vi "001_ZLG_CAN.vi"(11 "Queue Ref":T1={"UI"=refnum, "Message"=refnum, "Data"=refnum, "Caller"=refnum, "Name"="000 Common", "Data Path"=path "D:/NBT/01-Project/02-Processing/NBT-TestPlatform V2/NBT-TestPlatform V2.0.3/Config/NBT/NBT_V1.0.0/Project/0001_HZKD_ST01/00_DataSource/001_PLC/01_PLC", "Class Path"=path "", "SubPanel"=refnum, "Project Name"="", "MNT"="", "Title"="", "Data Source"=refnum, "Queue List"={}, "VI"=refnum, "UE"=refnum}) -> ()   [LabVIEW 2020]
doc: "001_ZLG_CAN.vi"
uses:
  Alin/QMH/000 Module Data Type.ctl
  Alin/QMH/Queue Message.ctl
  9999 SubVI/Global/Data Global/SDQ Data Type.ctl
  002 Driver/005 CAN/ZLG/ZLG_CAN_Channel.ctl
  002 Driver/005 CAN/ZLG/ZLG CAN.ctl
  002 Driver/005 CAN/ZLG/XNET_ZLG CAN/SubVIs/CAN/data_type/ZCAN_Transmit_Data.ctl
  <vilib>/Utility/miscctls.llb/LVMapReplaceAction.ctl
  002 Driver/005 CAN/ZLG/XNET_ZLG CAN/SubVIs/CAN/data_type/ZCAN_InitCAN_setting_CANET.ctl
  ba99fbad-406a-44a4-8ea9-c630dc189d5e.vi
  <vilib>/Utility/config.llb/Read Key (String).vi
  <vilib>/Utility/config.llb/Write Key (String).vi
  <vilib>/Utility/file.llb/Read Delimited Spreadsheet (string).vi
  <vilib>/Utility/file.llb/Write Delimited Spreadsheet (string).vi
  <vilib>/Utility/config.llb/NI_LVConfig.lvlib
panel:
  out "Name":string
  in  "Data Load":bool
  in  "ID":string(combo)
  out "Open":bool
  out "Read Delay(ms)":u32
  out "Write Delay(ms)":u32
  in  "Input":string
  in  "CAN Enable":bool
  out "Read":string[][](table) caption="单体电压排序(降序)"
  in  "Start Frame":u32=112 format="0x%08x"
  in  "Demo":string="{\"TIRC101_SV\":25.3,\"WorkMode_SV\":true}"
  in  "Multiple Parameter":string="{\"TIRC101_SV\":25.3,\"WorkMode_SV\":true}"
  in  "Write Test":bool
  out "Write Test":string[][](table) caption="单体电压排序(降序)"
  out "Write":string[][](table) caption="单体电压排序(降序)"
  out "Receive Frame":string
  out "Error":string
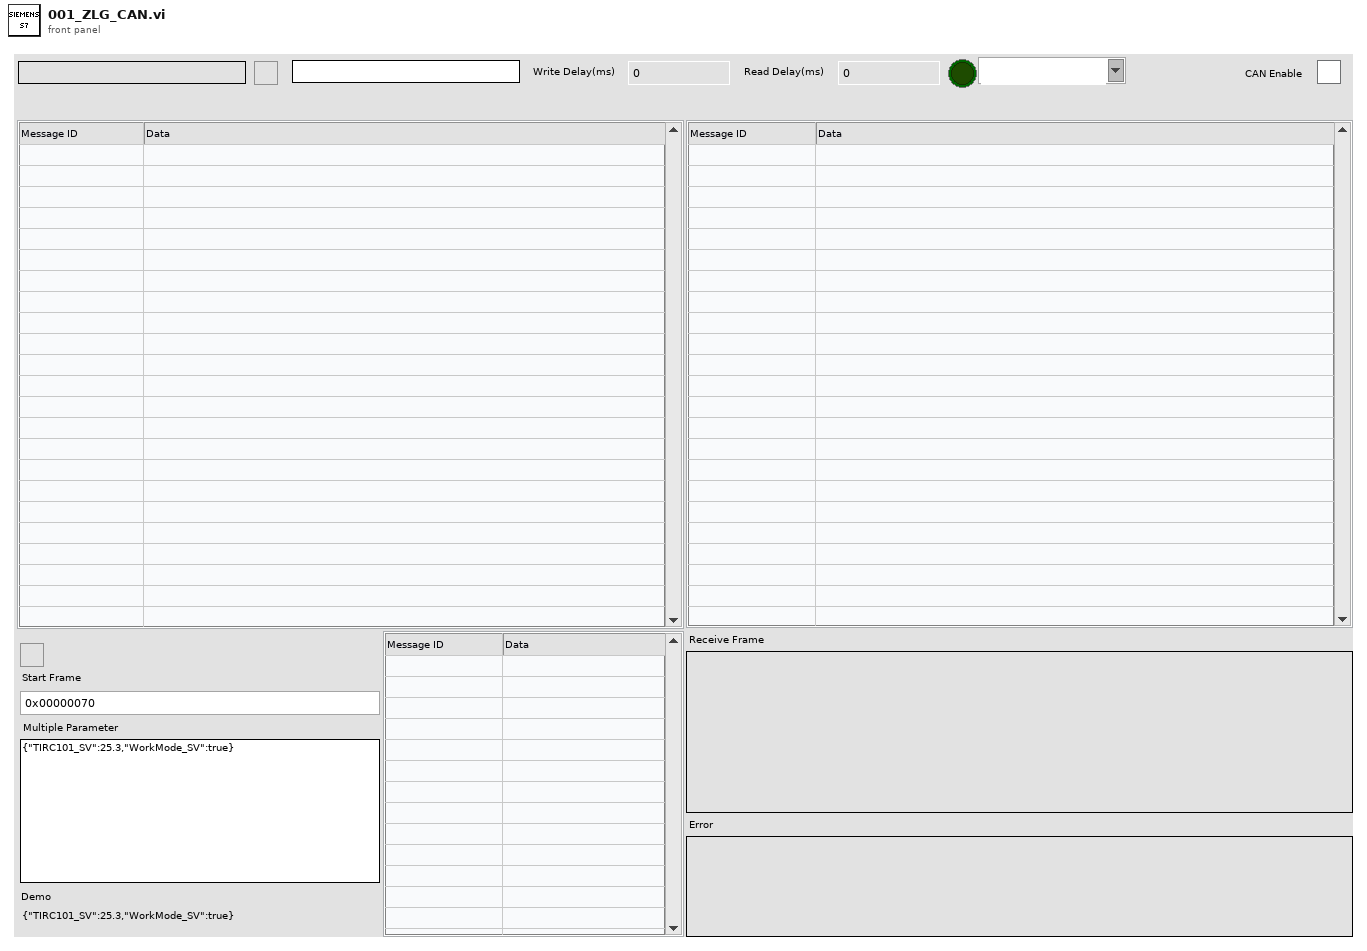
[diagram p1: front panel]
types:
  T1 = typedef "000 Module Data Type.ctl" = cluster{"UI":refnum<queue>, "Message":refnum<queue>, "Data":refnum<queue>, "Caller":refnum<queue>, "Name":string, "Data Path":path, "Class Path":path, "SubPanel":refnum<vi>, "Project Name":string, "MNT":string, "Title":string, "Data Source":refnum<queue>, "Queue List":map{string, refnum<queue>}, "VI":refnum<vi>, "UE":refnum<user-event>}
  T2 = typedef "SDQ Data Type.ctl" = cluster{"CAN Length":string, "CAN Name":string, "CAN ID":string, "CAN Type":string, "Test Item":string, "Byte Order":string, "Instruction":string, "Control Type":string, "Group":string, "Offset":dbl, "Coefficient":dbl, "Write Enable":bool, "Lable Type":string, "Key?":string, "Set Value":string, "Upper":dbl, "Lower":dbl, "Unit":string, "Formula":string, "Test Item Type":string, "Length":i32, "Address":string, "Name":string, "Identifier":string, "Data Type":string, "Enumerate?":string, "Enumerate List":string, "Data":string, "Source":string}
  T3 = typedef "ZLG_CAN_Channel.ctl" = cluster{"ChannelRef":u32, "DeviceRef":u32, "Reserved":u32, "CANModel":u32, "Index":u32, "CANChannel":u32, "TCPMode":u32, "LocalPort":u32, "RemotePort":u32, "IP":string, "Read?":bool, "Write?":bool}
  T4 = typedef "ZLG CAN.ctl" = cluster{"ID":string, "Name":string, "Length":i32, "Type":string, "Unit":string, "Upper":sgl, "Lower":sgl, "Set":i32, "Write Enable":bool, "Group":string, "Read Name":string, "CAN Fram Type":string, "CAN Message ID":string, "CAN Message Name":string, "CAN Byte Offset":i32, "CAN Bit Offset":i32, "CAN Message Length":i32, "Data":string}
  T5 = typedef "ZCAN_Transmit_Data.ctl" = cluster{"帧类型":u32, "帧格式":u32, "ID":u32, "数据长度":u8, "DATA":cluster{"CAN数据[0]":u8, "CAN数据[1]":u8, "CAN数据[2]":u8, "CAN数据[3]":u8, "CAN数据[4]":u8, "CAN数据[5]":u8, "CAN数据[6]":u8, "CAN数据[7]":u8}, "发送方式":u32}
  T6 = cluster{"Read Data":map{string, string}, "Open?":bool, "Queue Ref":T1, "Data":map{string, T2}, "Data List":T2[], "All Data":string[][], "Element":T2, "Title":string[], "Type":map{string, string}, "CAN":T3, "Delay":cluster{"Count Time(ms)":u32, "Delay Time(ms)":u32, "Next":string}, "CAN Data":map{string, T4}, "CAN Fram":map{string, map{string, T4}}, "ZCAN_Transmit_Data":T5, "CAN Element":u8[], "CAN Enable":bool, "dll Path":path}
  T7 = typedef "LVMapReplaceAction.ctl" = enum32{"Modify Entry only if found", "Add or Modify Entry", "Delete Entry"}
  T8 = typedef "ZCAN_InitCAN_setting_CANET.ctl" = cluster{"tcp_type":u32, "work_port":u32, "local_port":u32, "IP":string}
  T9 = typedef "NI_LVConfig.lvlib/Config Data RefNum.ctl" = refnum<k1>
  T10 = cluster{"Name":string, "Type":map{string, string}}
  T11 = cluster{u32, u8, u8, u8, u8, cluster{"[0]":u8, "[1]":u8, "[2]":u8, "[3]":u8, "[4]":u8, "[5]":u8, "[6]":u8, "[7]":u8}, u64}[]
  T12 = cluster{"CAN Element[0]":u8, "CAN Element[1]":u8, "CAN Element[2]":u8, "CAN Element[3]":u8, "CAN Element[4]":u8, "CAN Element[5]":u8, "CAN Element[6]":u8, "CAN Element[7]":u8}
  T13 = cluster{"CAN数据[0]":u8, "CAN数据[1]":u8, "CAN数据[2]":u8, "CAN数据[3]":u8, "CAN数据[4]":u8, "CAN数据[5]":u8, "CAN数据[6]":u8, "CAN数据[7]":u8}
  T14 = cluster{u32, "数据长度":u8, u8, u8, u8, "DATA":cluster{"CAN数据[0]":u8, "CAN数据[1]":u8, "CAN数据[2]":u8, "CAN数据[3]":u8, "CAN数据[4]":u8, "CAN数据[5]":u8, "CAN数据[6]":u8, "CAN数据[7]":u8}, "发送方式":u32}
  T15 = typedef "eventvkey.ctl" = enum16{"ASCII", "Enter", "Return", "Shift", "Ctrl", "Alt", "Cmd", "Opt", "Caps", "NumLock", "Clear", "Break", "Up", "Down", "Left", "Right", "Insert", "Delete", "Home", "End", "PageUp", "PageDown", "Escape", "Help", "Pause", "ScrollLock", "F1", "F2", "F3", "F4", "F5", "F6", "F7", "F8", "F9", "F10", "F11", "F12", "F13", "F14", "F15", "F16", "F17", "F18", "F19", "F20", "F21", "F22", "F23", "F24", "Play", "VolumeUp", "VolumeDown", "Mute", "Two Byte Char"}
  T16 = cluster{"Shift":bool, "Ctrl":bool, "Alt":bool, "Cmd":bool, "Opt":bool}
  T17 = cluster{"Queue List":map{string, refnum<queue>}, "Active Panel":string, "Queue":T1, "Active Row":i32, "All Data":string[][]}
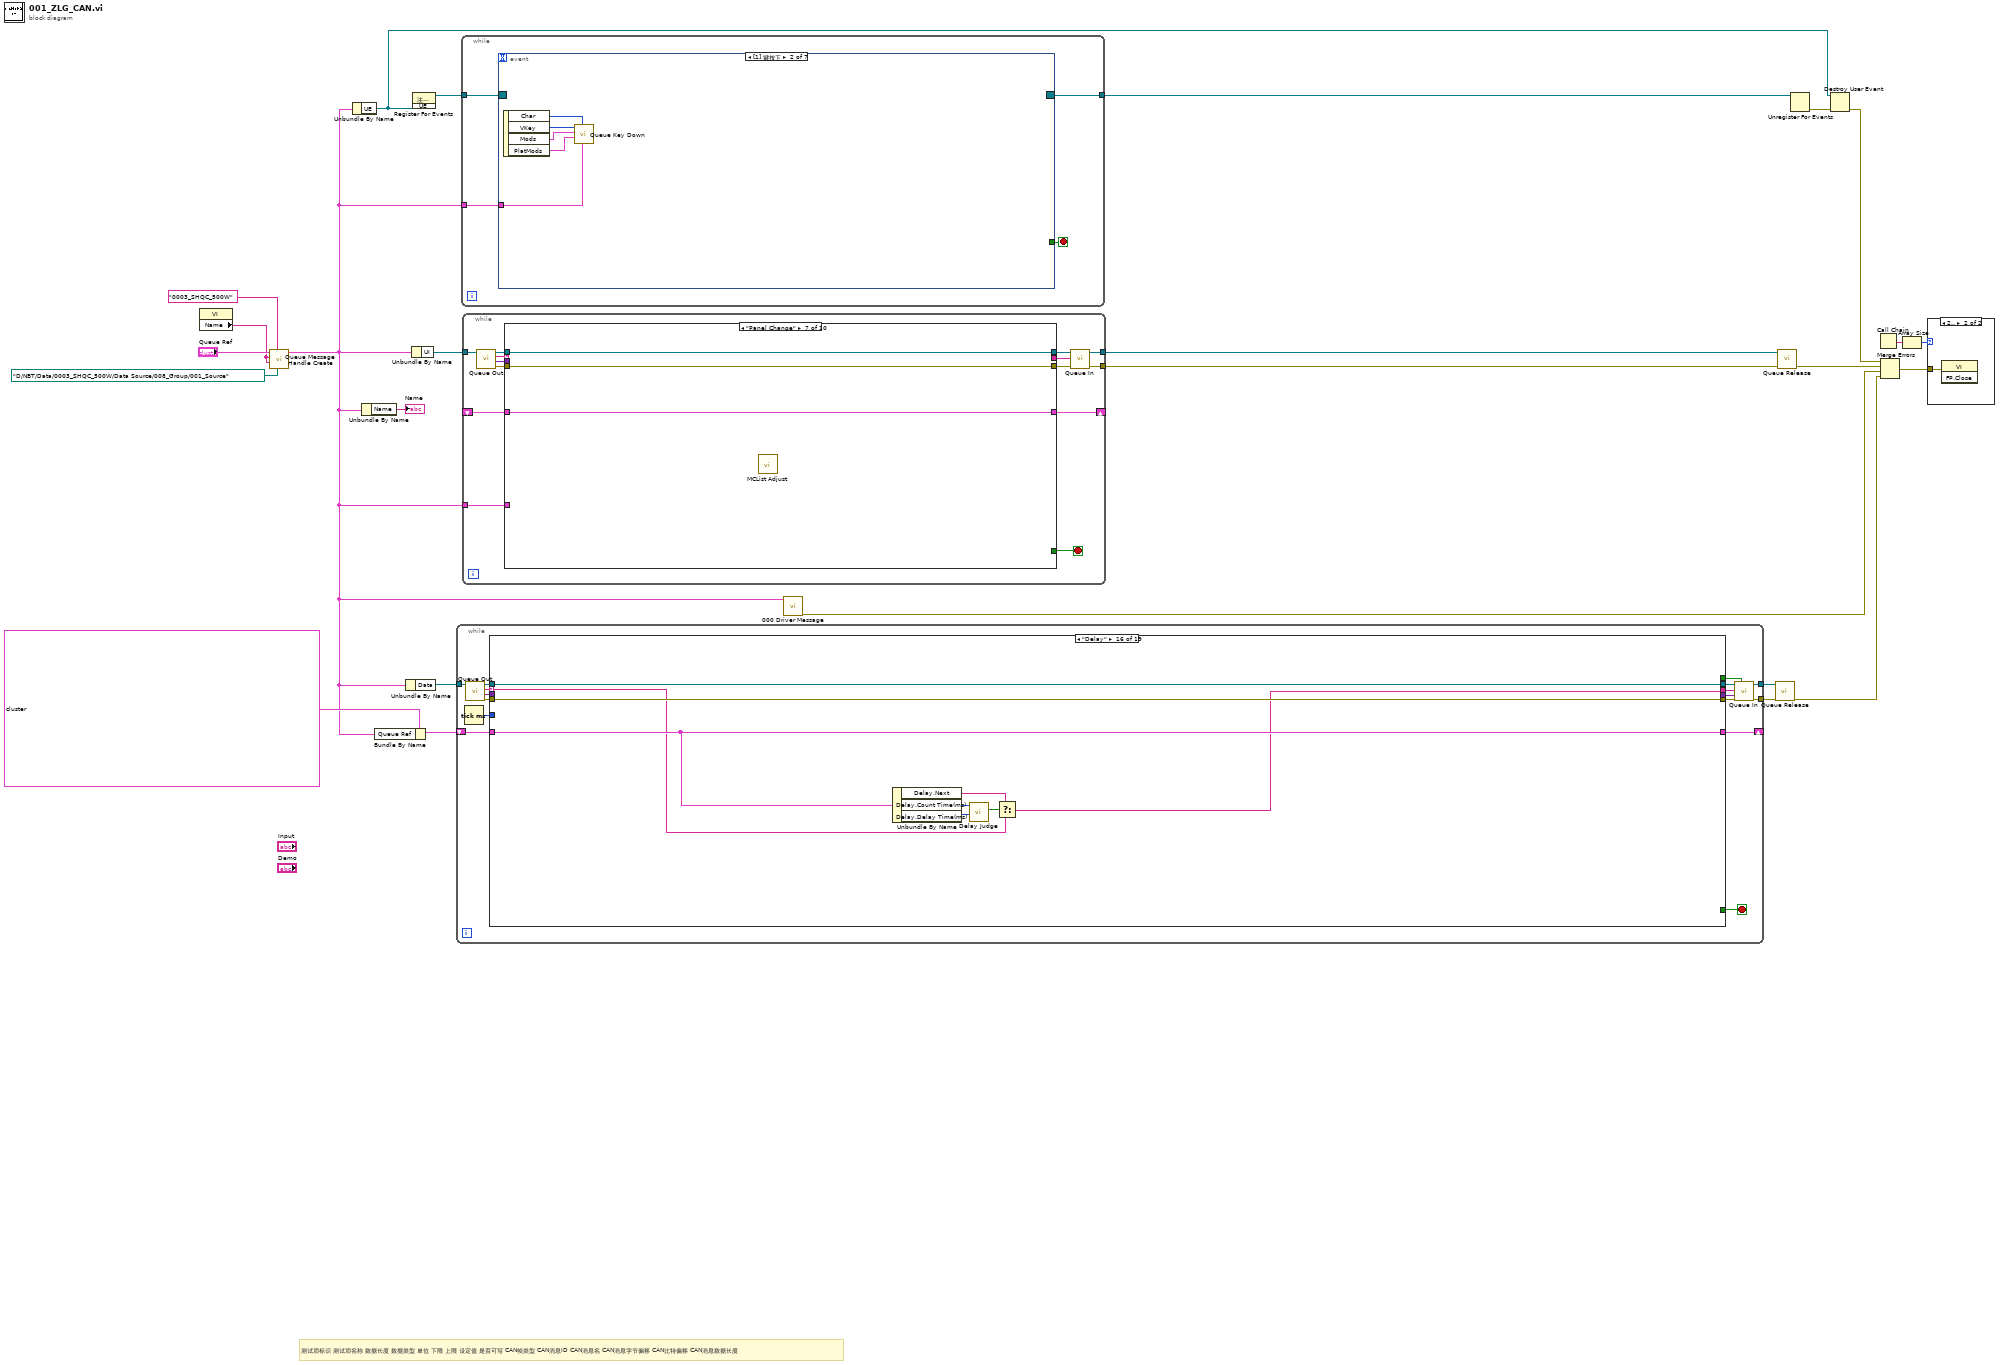
[diagram p0: block diagram]
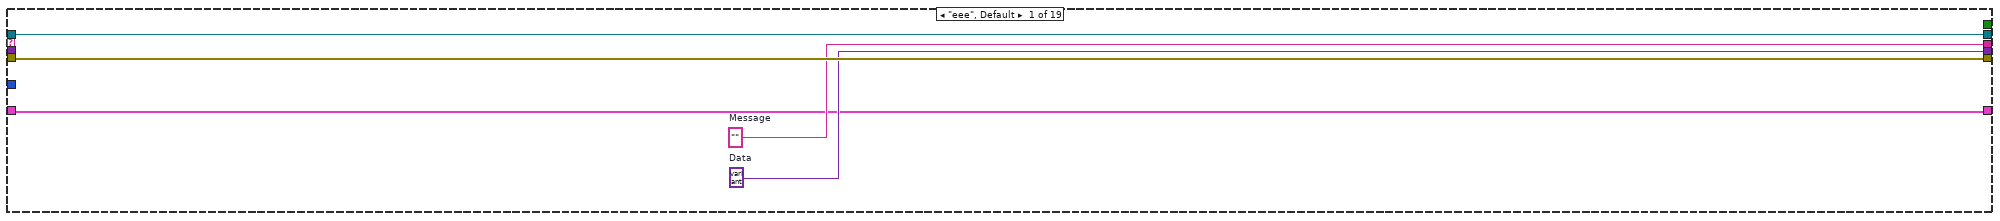
[diagram p2: hidden frame]
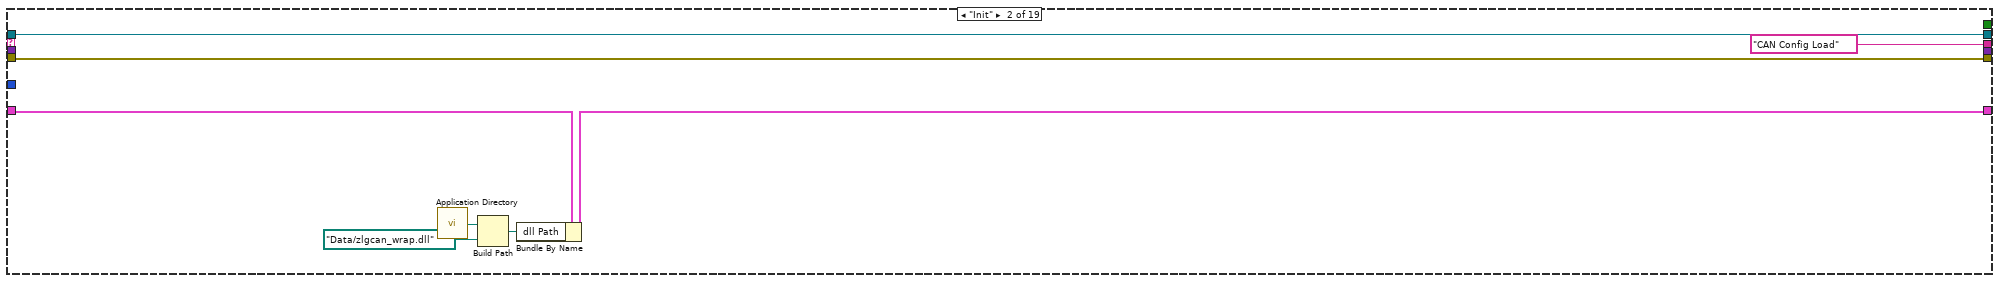
[diagram p3: hidden frame]
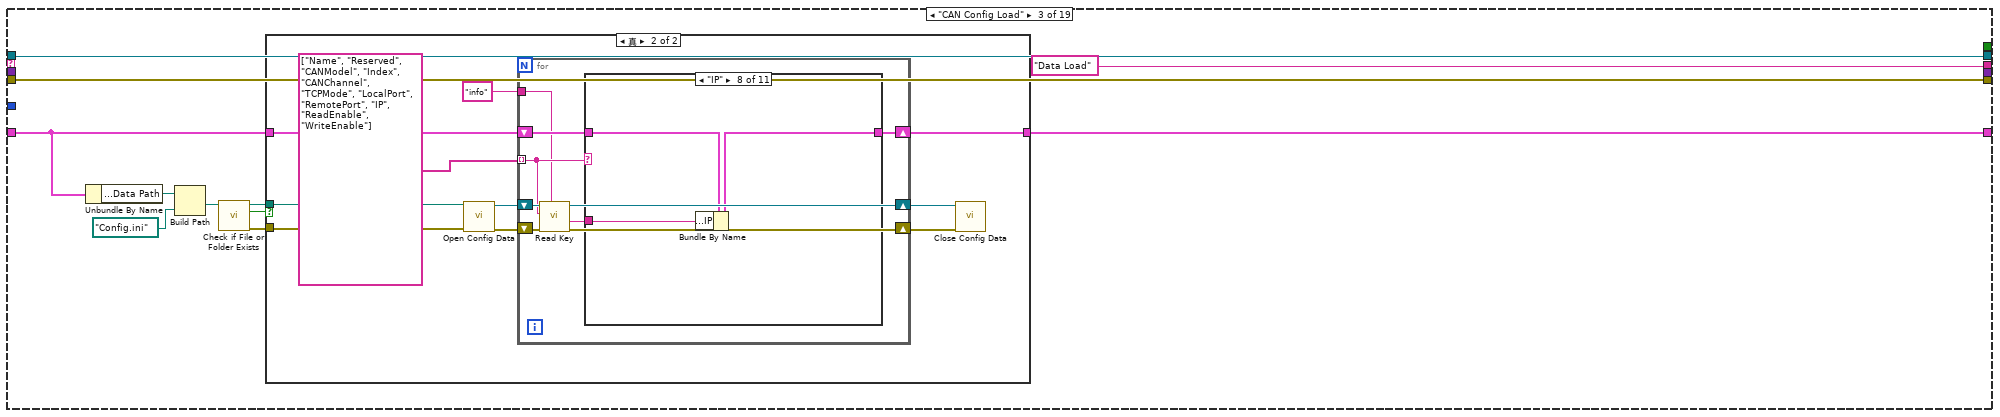
[diagram p4: hidden frame]
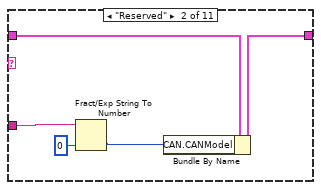
[diagram p7: hidden frame]
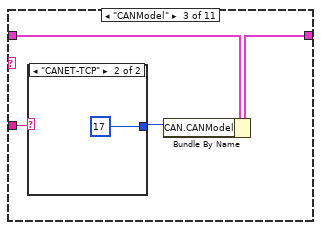
[diagram p8: hidden frame]
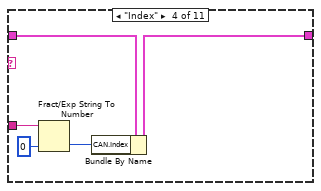
[diagram p10: hidden frame]
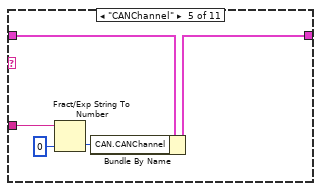
[diagram p11: hidden frame]
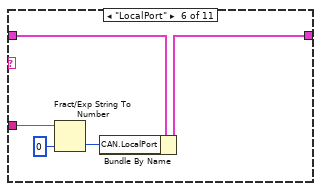
[diagram p12: hidden frame]
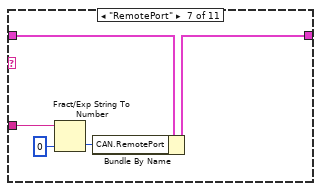
[diagram p13: hidden frame]
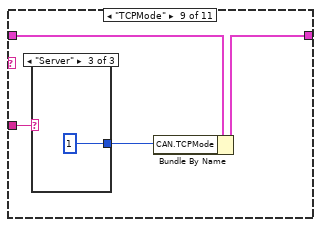
[diagram p14: hidden frame]
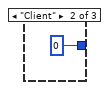
[diagram p16: hidden frame]
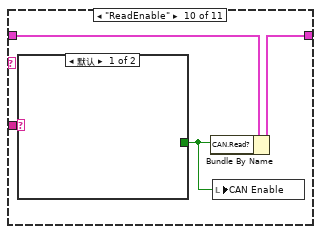
[diagram p17: hidden frame]
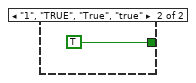
[diagram p18: hidden frame]
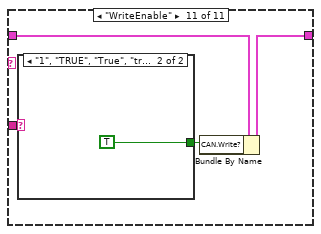
[diagram p19: hidden frame]
diagram:
  # "测试项标识\t测试项名称\t数据长度\t数据类型\t单位\t下限\t上限\t设定值\t是否可写\tCAN帧类型\tCAN消息ID\tCAN消息名\tCAN消息字节偏移\tCAN比特偏移\tCAN消息数据长度"
  n1 = property class="VI"() -> ("Name"=w4:string)  [unwired: 2 in, 2 out]
  n2 = call "Queue Message Handle Create.vi"("Data Path"=path "D:/NBT/Data/0003_SHQC_500W/Data Source/008_Group/001_Source", "Project Name"="0003_SHQC_500W", "Name"=w4, "Title"=w4, "Queue Ref In"="Queue Ref") -> ("Queue Ref Out"=w2:T1)  [unwired: 5 in, 1 out]
  n3 = Unbundle By Name(w2) -> ("UE"=w12:refnum<user-event>)
  n4 = Unbundle By Name(w2) -> ("Name"=→"Name":string)
  n5 = Bundle By Name(cluster=T6 {"Read Data"={}, "Open?"=FALSE, "Queue Ref"={"UI"=refnum, "Message"=refnum, "Data"=refnum, "Caller"=refnum, "Name"="", "Data Path"=path "", "Class Path"=path "", "SubPanel"=refnum, "Project Name"="", "MNT"="", "Title"="", "Data Source"=refnum, "Queue List"={}, "VI"=refnum, "UE"=refnum}, "Data"={}, "Data List"=[], "All Data"=[], "Element"={"CAN Length"="", "CAN Name"="", "CAN ID"="", "CAN Type"="", "Test Item"="", "Byte Order"="", "Instruction"="", "Control Type"="", "Group"="", "Offset"=0.0, "Coefficient"=0.0, "Write Enable"=FALSE, "Lable Type"="", "Key?"="", "Set Value"="", "Upper"=0.0, "Lower"=0.0, "Unit"="", "Formula"="", "Test Item Type"="", "Length"=0, "Address"="", "Name"="", "Identifier"="", "Data Type"="", "Enumerate?"="", "Enumerate List"="", "Data"="", "Source"=""}, "Title"=[], "Type"={}, "CAN"={"ChannelRef"=0, "DeviceRef"=0, "Reserved"=0, "CANModel"=17, "Index"=0, "CANChannel"=0, "TCPMode"=0, "LocalPort"=8000, "RemotePort"=4001, "IP"="192.168.0.178", "Read?"=FALSE, "Write?"=FALSE}, "Delay"={"Count Time(ms)"=250, "Delay Time(ms)"=50, "Next"="Write,Read,Delay"}, "CAN Data"={}, "CAN Fram"={}, "ZCAN_Transmit_Data"={"帧类型"=0, "帧格式"=0, "ID"=0, "数据长度"=8, "DATA"={"CAN数据[0]"=0, "CAN数据[1]"=0, "CAN数据[2]"=0, "CAN数据[3]"=0, "CAN数据[4]"=0, "CAN数据[5]"=0, "CAN数据[6]"=0, "CAN数据[7]"=0}, "发送方式"=0}, "CAN Element"=[0, 0, 0, 0, 0, 0, 0, 0], "CAN Enable"=FALSE, "dll Path"=path ""}, "Queue Ref"=w2) -> (w7:T6)
  n6 = Unbundle By Name(w2) -> ("Data"=w9:refnum<queue>)
  n7 = Unbundle By Name(w2) -> ("UI"=w18:refnum<queue>)
  n8 = register-events(w12) -> (reference out=w13:refnum<event-registration>)  [unwired: 2 in, 1 out]
  n9 = while {
    tunnel: w9 -> [w38]
    tunnel: [w35] -> w5
    tunnel: [w34] -> w6
    shift-right: [w29] -> _
    shift-left: w7 -> [w30]
    stop <- w41 stop-if-true
    n10 = Tick Count (ms)() -> (millisecond timer value=w26:u32)
    n11 = call "Queue Out.vi"("Queue In"=w38) -> ("error out"=w40:errorcluster, "Data"=w39:variant, "Message"=w27:string, "Queue Out"=w37:refnum<queue>)  [unwired: 6 in, 1 out]
    n12 = case shown="\"Delay\"" w27 {
      selector: w27 -> [_ _ _ _ _ _ _ _ _ _ _ _ _ _ _ w748 _ _ _]
      tunnel: w37 -> [w46 w54 w65 w145 w172 w307 w331 w365 w377 w406 w426 w474 w508 w663 w741 w755 w762 w767 w771]
      tunnel: w40 -> [w45 w53 w64 w144 w171 w306 w330 w364 w376 w405 w425 w473 w507 w662 w740 w754 w761 w765 w772]
      tunnel: [w46 w54 w65 w145 w172 w307 w331 w365 w377 w403 w426 w474 w508 w663 w741 w755 w762 w766 w771] -> w36
      tunnel: [w45 w53 w64 w144 w171 w306 w330 w364 w376 w404 w425 w473 w507 w662 w740 w754 w761 w764 w772] -> w33
      tunnel: [w44 "CAN Config Load" ("Message") "Data Load" ("Message") _ "Close,Open" ("Message") "Data Load" ("Message") "Send" ("Message") "Read" ("Message") _ w401 w424 "Delay" ("Message") w506 w661 _ w747 _ "Close,Quit" _] -> w32
      tunnel: [_ _ _ _ _ _ _ _ _ _ _ _ _ _ _ _ _ _ TRUE] -> w41
      tunnel: [w43 _ _ _ _ _ _ _ _ w400 w421 _ w504 w659 _ _ _ _ _] -> w31
      tunnel: w39 -> [_ _ _ w138 _ w304 _ _ _ _ _ _ _ _ _ _ w758 _ _]
      tunnel: [w42 w48 w56 w137 w160 w298 w322 w359 w375 w378 w422 w471 w494 w656 w735 w749 w760 w763 w769] -> w29
      tunnel: w30 -> [w42 w51 w57 w140 w164 w305 w326 w352 w375 w402 w419 w471 w499 w656 w739 w749 w760 w763 w769]
      tunnel: [_ _ _ _ _ _ _ _ _ _ w423 _ w505 w660 _ _ _ _ _] -> w28
      tunnel: w26 -> [_ _ _ _ _ _ _ _ _ _ w420 _ w496 w653 _ _ _ _ _]
      frame "eee", Default {
        w43 = variant  # Data
        w44 = ""  # Message
      }
      frame "Init" {
        n13 = call <vilib>:"Application Directory.vi"() -> ("Application Directory"=w50:path)
        n14 = Build Path(base path=w50, name or relative path=path "Data/zlgcan_wrap.dll" ("名称或相对路径")) -> (appended path=w47:path)
        n15 = Bundle By Name(cluster=w51, "dll Path"=w47) -> (w48:T6)
      }
      frame "CAN Config Load" {
        n16 = Unbundle By Name(w57) -> ("Queue Ref.Data Path"=w63:path)
        n17 = Build Path(base path=w63, name or relative path=path "Config.ini" ("名称或相对路径")) -> (appended path=w61:path)
        n18 = call <vilib>:"Check if File or Folder Exists.vi"("path"=w61) -> ("error out"=w58:errorcluster, "file or folder exists?"=w60:bool, "dup path"=w59:path)  [unwired: 8 in]
        n19 = case shown="真" w60 {
          tunnel: w59 -> [_ w71]
          tunnel: w58 -> [_ w72]
          tunnel: w57 -> [w66 w69]
          tunnel: [w66 w68] -> w56
          frame False {
          }
          frame True {
            n20 = call <vilib>:"Open Config Data.vi"("error in (no error)"=w72, "configuration file path"=w71) -> ("error out"=w75:errorcluster, "refnum"=w76:T9)  [unwired: 7 in, 1 out]
            n21 = for {
              shift-right: [w83] -> w74
              shift-left: w76 -> [w85]
              shift-right: [w82] -> w73
              shift-left: w75 -> [w84]
              tunnel: string[] ["Name", "Reserved", "CANModel", "Index", "CANChannel", "TCPMode", "LocalPort", "RemotePort", "IP", "ReadEnable", "WriteEnable"] -> [w81] mode=indexing
              shift-right: [w79] -> w68
              shift-left: w69 -> [w80]
              tunnel: "info" ("section") -> [w77]
              n22 = call-poly <vilib>:"Read Key.vi"("section"=w77, "error in (no error)"=w84, "key"=w81, "refnum"=w85) -> ("error out"=w82:errorcluster, "value"=w78:string, "refnum out"=w83:T9)  [unwired: 4 in, 1 out]
              n23 = case shown="\"IP\"" w81 {
                tunnel: w80 -> [w86 w91 w95 w101 w106 w111 w116 w119 w123 w129 w134]
                tunnel: [w86 w90 w94 w100 w105 w110 w115 w118 w122 w128 w133] -> w79
                tunnel: w78 -> [_ w88 w93 w99 w104 w109 w114 w117 w121 w127 w132]
                frame Default {
                }
                frame "Reserved" {
                  n24 = Fract/Exp String To Number(string=w88, default (0 dbl)=u32 0 ("CAN.Reserved")) -> (number=w87:u32)  [unwired: 2 in, 1 out]
                  n25 = Bundle By Name(cluster=w91, "CAN.CANModel"=w87) -> (w90:T6)
                }
                frame "CANModel" {
                  n26 = case shown="\"CANET-TCP\"" w93 {
                    tunnel: [_ u32 17 ("CAN.CANModel")] -> w92
                    frame Default {
                    }
                    frame "CANET-TCP" {
                    }
                  }
                  n27 = Bundle By Name(cluster=w95, "CAN.CANModel"=w92) -> (w94:T6)
                }
                frame "Index" {
                  n28 = Fract/Exp String To Number(string=w99, default (0 dbl)=u32 0 ("CAN.Reserved")) -> (number=w97:u32)  [unwired: 2 in, 1 out]
                  n29 = Bundle By Name(cluster=w101, "CAN.Index"=w97) -> (w100:T6)
                }
                frame "CANChannel" {
                  n30 = Fract/Exp String To Number(string=w104, default (0 dbl)=u32 0 ("CAN.Reserved")) -> (number=w102:u32)  [unwired: 2 in, 1 out]
                  n31 = Bundle By Name(cluster=w106, "CAN.CANChannel"=w102) -> (w105:T6)
                }
                frame "LocalPort" {
                  n32 = Fract/Exp String To Number(string=w109, default (0 dbl)=u32 0 ("CAN.Reserved")) -> (number=w107:u32)  [unwired: 2 in, 1 out]
                  n33 = Bundle By Name(cluster=w111, "CAN.LocalPort"=w107) -> (w110:T6)
                }
                frame "RemotePort" {
                  n34 = Fract/Exp String To Number(string=w114, default (0 dbl)=u32 0 ("CAN.Reserved")) -> (number=w112:u32)  [unwired: 2 in, 1 out]
                  n35 = Bundle By Name(cluster=w116, "CAN.RemotePort"=w112) -> (w115:T6)
                }
                frame "IP" {
                  n36 = Bundle By Name(cluster=w119, "CAN.IP"=w117) -> (w118:T6)
                }
                frame "TCPMode" {
                  n37 = case shown="\"Server\"" w121 {
                    tunnel: [_ u32 0 ("CAN.TCPMode") u32 1 ("CAN.TCPMode")] -> w120
                    frame Default {
                    }
                    frame "Client" {
                    }
                    frame "Server" {
                    }
                  }
                  n38 = Bundle By Name(cluster=w123, "CAN.TCPMode"=w120) -> (w122:T6)
                }
                frame "ReadEnable" {
                  n39 = case shown="默认" w127 {
                    tunnel: [_ TRUE] -> w126
                    frame Default {
                    }
                    frame "1", "TRUE", "True", "true" {
                    }
                  }
                  n40 = Bundle By Name(cluster=w129, "CAN.Read?"=w126) -> (w128:T6)
                  n41 = local write "CAN Enable"(w126) -> ()
                }
                frame "WriteEnable" {
                  n42 = case shown="\"1\", \"TRUE\", \"True\", \"true\"" w132 {
                    tunnel: [_ TRUE] -> w131
                    frame Default {
                    }
                    frame "1", "TRUE", "True", "true" {
                    }
                  }
                  n43 = Bundle By Name(cluster=w134, "CAN.Write?"=w131) -> (w133:T6)
                }
              }
            }
            n44 = call <vilib>:"Close Config Data.vi"("error in (no error)"=w73, "refnum"=w74) -> ()  [unwired: 8 in, 2 out]
          }
        }
      }
      frame "CAN Enable" {
        n45 = Unbundle By Name(w140) -> ("Queue Ref.Data Path"=w143:path)
        n46 = Build Path(base path=w143, name or relative path=path "Config.ini" ("名称或相对路径")) -> (appended path=w141:path)
        n47 = call <vilib>:"Check if File or Folder Exists.vi"("path"=w141) -> ("file or folder exists?"=w136:bool, "dup path"=w139:path)  [unwired: 8 in, 1 out]
        n48 = Bundle By Name(cluster=w140, "CAN.Read?"=w136) -> (w137:T6)
        n49 = case shown="真" w136 {
          tunnel: w139 -> [_ w158]
          tunnel: w138 -> [_ w153]
          frame False {
          }
          frame True {
            n50 = Variant To Data(type=FALSE, Variant=w153) -> (data=w151:bool)  [unwired: 1 in, 1 out]
            n51 = call <vilib>:"Open Config Data.vi"("configuration file path"=w158) -> ("error out"=w156:errorcluster, "refnum"=w157:T9)  [unwired: 8 in, 1 out]
            n52 = Select(t="1", s=w151, f="0") -> (s? t:f=w146:string)
            n53 = call-poly <vilib>:"Write Key.vi"("section"="info", "error in (no error)"=w156, "value"=w146, "key"="ReadEnable", "refnum"=w157) -> ("error out"=w155:errorcluster, "refnum out"=w154:T9)  [unwired: 4 in, 1 out]
            n54 = call <vilib>:"Close Config Data.vi"("error in (no error)"=w155, "refnum"=w154) -> ()  [unwired: 8 in, 2 out]
          }
        }
      }
      frame "Data Load" {
        n55 = Unbundle By Name(w164) -> ("Queue Ref.Data Path"=w170:path)
        n56 = Build Path(base path=w170, name or relative path=path "CAN.csv" ("名称或相对路径")) -> (appended path=w168:path)
        n57 = call <vilib>:"Check if File or Folder Exists.vi"("path"=w168) -> ("error out"=w165:errorcluster, "file or folder exists?"=w167:bool, "dup path"=w166:path)  [unwired: 8 in]
        n58 = case shown="真" w167 {
          tunnel: w166 -> [_ w200]
          tunnel: w165 -> [_ w201]
          tunnel: w164 -> [w191 w194]
          tunnel: [w191 w193] -> w159
          tunnel: LVMapReplaceAction."Add or Modify Entry" ("操作") -> [_ w192]
          frame False {
          }
          frame True {
            n59 = call-poly <vilib>:"Read Delimited Spreadsheet.vi"("file path (dialog if empty)"=w200, "error in (no error)"=w201, "delimiter (\\t)"="," ("delimiter (\\t)")) -> ("all rows"=w198:string[][])  [unwired: 7 in, 5 out]
            n60 = Delete From Array(array=w198, length=1 ("长度"), index (row)=0 ("索引 (行)")) -> (array with subset deleted=w195:string[][])  [unwired: 1 in, 1 out]
            n61 = in-place {
              in-place-border: w195 -> [w204]
              in-place-border: w192 -> [w205]
              n62 = in-place-cluster #1(w194) -> ("CAN Data"=w207:map{string, T4})
              n63 = Index Array(array=w204, index (col)=0 ("禁用的索引 (列)")) -> (element=w202:string[])  [unwired: 1 in]
              n64 = property on="ID" class="CmbBox"("Strings[]"=w202) -> ()  [unwired: 2 in, 2 out]
              n65 = for {
                tunnel: w204 -> [w209] mode=indexing
                shift-right: [w211] -> w206
                shift-left: w207 -> [w212]
                tunnel: w205 -> [w210]
                n66 = Index Array(array=w209) -> (element=w208:string)  [unwired: 1 in]
                n67 = in-place {
                  in-place-border: w209 -> [w216]
                  in-place-border: w210 -> [w213]
                  n68 = in-place-map #2(w212, w208) -> (w215:T4)  [unwired: 1 in, 1 out]
                  n69 = for {
                    tunnel: w216 -> [w218] mode=indexing
                    shift-right: [w219] -> w214
                    shift-left: w215 -> [w220]
                    i -> [w217]
                    n70 = case shown="8" w217 {
                      tunnel: [w222 w225 w230 w233 w236 w241 w246 w251 w256 w260 w263 w266 w269 w272 w277 w282 w287 w289] -> w219
                      tunnel: w220 -> [w223 w226 w231 w234 w237 w242 w247 w252 w257 w261 w264 w267 w270 w273 w278 w283 w288 w289]
                      tunnel: w218 -> [w221 w224 w229 w232 w235 w240 w245 w250 w255 w259 w262 w265 w268 w271 w276 w281 w286 _]
                      frame 0, Default {
                        # "ID"
                        n71 = Bundle By Name(cluster=w223, "ID"=w221) -> (w222:T4)
                      }
                      frame 1 {
                        # "Name"
                        n72 = Bundle By Name(cluster=w226, "Name"=w224) -> (w225:T4)
                      }
                      frame 2 {
                        # "Length"
                        n73 = Fract/Exp String To Number(string=w229, default (0 dbl)=0 ("Length")) -> (number=w227:i32)  [unwired: 2 in, 1 out]
                        n74 = Bundle By Name(cluster=w231, "Length"=w227) -> (w230:T4)
                      }
                      frame 3 {
                        # "Type"
                        n75 = Bundle By Name(cluster=w234, "Type"=w232) -> (w233:T4)
                      }
                      frame 4 {
                        # "Unit"
                        n76 = Bundle By Name(cluster=w237, "Unit"=w235) -> (w236:T4)
                      }
                      frame 5 {
                        # "Upper"
                        n77 = Fract/Exp String To Number(string=w240, default (0 dbl)=sgl 0.0 ("Length")) -> (number=w238:sgl)  [unwired: 2 in, 1 out]
                        n78 = Bundle By Name(cluster=w242, "Upper"=w238) -> (w241:T4)
                      }
                      frame 6 {
                        # "Lower"
                        n79 = Fract/Exp String To Number(string=w245, default (0 dbl)=sgl 0.0 ("Length")) -> (number=w243:sgl)  [unwired: 2 in, 1 out]
                        n80 = Bundle By Name(cluster=w247, "Lower"=w243) -> (w246:T4)
                      }
                      frame 7 {
                        # "Set"
                        n81 = Fract/Exp String To Number(string=w250, default (0 dbl)=0 ("Length")) -> (number=w248:i32)  [unwired: 2 in, 1 out]
                        n82 = Bundle By Name(cluster=w252, "Set"=w248) -> (w251:T4)
                      }
                      frame 8 {
                        # "Write Enable"
                        n83 = To Lower Case(string=w255) -> (all lower case string=w253:string)
                        n84 = case shown="默认" w253 {
                          tunnel: [_ TRUE] -> w254
                          frame Default {
                          }
                          frame "1", "true" {
                          }
                        }
                        n85 = Bundle By Name(cluster=w257, "Write Enable"=w254) -> (w256:T4)
                      }
                      frame 9 {
                        # "Group"
                        n86 = Bundle By Name(cluster=w261, "Group"=w259) -> (w260:T4)
                      }
                      frame 10 {
                        # "Group"
                        n87 = Bundle By Name(cluster=w264, "Read Name"=w262) -> (w263:T4)
                      }
                      frame 11 {
                        # "CAN Fram Type"
                        n88 = Bundle By Name(cluster=w267, "CAN Fram Type"=w265) -> (w266:T4)
                      }
                      frame 12 {
                        # "CAN Message ID"
                        n89 = Bundle By Name(cluster=w270, "CAN Message ID"=w268) -> (w269:T4)
                      }
                      frame 13 {
                        # "CAN Message Name"
                        n90 = Bundle By Name(cluster=w273, "CAN Message Name"=w271) -> (w272:T4)
                      }
                      frame 14 {
                        # "CAN Byte Offset"
                        n91 = Fract/Exp String To Number(string=w276, default (0 dbl)=0 ("Length")) -> (number=w274:i32)  [unwired: 2 in, 1 out]
                        n92 = Bundle By Name(cluster=w278, "CAN Byte Offset"=w274) -> (w277:T4)
                      }
                      frame 15 {
                        # "CAN Bit Offset"
                        n93 = Fract/Exp String To Number(string=w281, default (0 dbl)=0 ("Length")) -> (number=w279:i32)  [unwired: 2 in, 1 out]
                        n94 = Bundle By Name(cluster=w283, "CAN Bit Offset"=w279) -> (w282:T4)
                      }
                      frame 16 {
                        # "CAN Message Length"
                        n95 = Fract/Exp String To Number(string=w286, default (0 dbl)=0 ("Length")) -> (number=w284:i32)  [unwired: 2 in, 1 out]
                        n96 = Bundle By Name(cluster=w288, "CAN Message Length"=w284) -> (w287:T4)
                      }
                      frame 17.. {
                      }
                    }
                  }
                  n97 = in-place-map #2(w214, w213) -> (w211:map{string, T4})  [unwired: 2 out]
                }
              }
              n98 = in-place-cluster #1("CAN Data"=w206) -> (w193:T6)
            }
          }
        }
        n99 = Unbundle By Name(w159) -> ("CAN Data"=w161:map{string, T4})
        n100 = for {
          tunnel: w161 -> [w175] mode=indexing
          shift-right: [w177] -> w160
          shift-left: w159 -> [w178]
          n101 = Unbundle By Name(w175) -> ("CAN.CAN Message ID"=w176:string, "CAN"=w174:T4)
          n102 = in-place {
            in-place-border: w176 -> [w181]
            in-place-border: w174 -> [w180]
            in-place-border: LVMapReplaceAction."Add or Modify Entry" ("操作") -> [w179]
            n103 = in-place-cluster #3(w178) -> ("CAN Fram"=w183:map{string, map{string, T4}})
            n104 = in-place {
              in-place-border: w180 -> [w186]
              in-place-border: w179 -> [w184]
              n105 = in-place-map #4(w183, w181) -> (w188:map{string, T4})  [unwired: 1 in, 1 out]
              n106 = Unbundle By Name(w186) -> ("ID"=w185:string)
              n107 = in-place {
                in-place-border: w186 -> [w190]
                in-place-border: w184 -> [w189]
                n108 = in-place-map #5(w188, w185) -> ()  [unwired: 1 in, 2 out]
                n109 = in-place-map #5(w190, w189) -> (w187:map{string, T4})  [unwired: 2 out]
              }
              n110 = in-place-map #4(w187, w184) -> (w182:map{string, map{string, T4}})  [unwired: 2 out]
            }
            n111 = in-place-cluster #3("CAN Fram"=w182) -> (w177:T6)
          }
        }
      }
      frame "Data Save" {
        n112 = in-place {
          in-place-border: w304 -> [w319]
          n113 = in-place-cluster #6(w305) -> ("Element"=w318:T2)
          n114 = Variant To Data(type=w318, Variant=w319) -> (data=w317:T2)  [unwired: 1 in, 1 out]
          n115 = in-place-cluster #6("Element"=w317) -> (w303:T6)
        }
        n116 = Unbundle By Name(w303) -> ("Element.Identifier"=w302:string, "Element"=w301:T2)
        n117 = in-place {
          in-place-border: w302 -> [w315]
          in-place-border: w301 -> [w314]
          in-place-border: [w313] -> w299
          n118 = in-place-cluster #7(w303) -> ("Data"=w316:map{string, T2})
          n119 = Insert Into Map(map in=w316, key=w315, value=w314) -> (map out=w313:map{string, T2})  [unwired: 2 out]
          n120 = in-place-cluster #7("Data"=w313) -> (w298:T6)
        }
        n121 = Unbundle By Name(w298) -> ("All Data"=w300:string[][])
        n122 = for {
          tunnel: w300 -> [w311] mode=indexing
          tunnel: w299 -> [w312]
          tunnel: [w308] -> w296 mode=indexing
          n123 = Index Array(array=w311) -> (element=w310:string)  [unwired: 1 in]
          n124 = Look In Map(map=w312, key=w310) -> (value=w309:T2)  [unwired: 1 in, 1 out]
          n125 = call "File to Element.vi"("Element In"=w309) -> ("Data Out"=w308:string[])  [unwired: 9 in, 1 out]
        }
        n126 = Unbundle By Name(w298) -> ("Queue Ref.Data Path"=w292:path, "Title"=w297:string[])
        n127 = Build Array (concatenate)(w297, w296) -> (w295:string[][])
        n128 = Build Path(base path=w292, name or relative path=path "Data.csv" ("名称或相对路径")) -> (appended path=w290:path)
        n129 = call-poly <vilib>:"Write Delimited Spreadsheet.vi"("file path (dialog if empty)"=w290, "2D data"=w295, "delimiter (\\t)"="," ("delimiter (\\t)")) -> ()  [unwired: 11 in, 2 out]
      }
      frame "Data Monitor" {
        n130 = Unbundle By Name(w326) -> ("Data"=w327:map{string, T2}, "Queue Ref.Name"=w320:string)
        n131 = for {
          tunnel: w327 -> [w337] mode=indexing
          shift-right: [w338] -> w325
          shift-left: w326 -> [w339]
          tunnel: w320 -> [w336]
          n132 = in-place {
            in-place-border: w337 -> [w343]
            in-place-border: w336 -> [w340]
            n133 = in-place-cluster #8(w339) -> ("Data"=w346:map{string, T2})
            n134 = Unbundle By Name(w343) -> ("Data"=w344:T2)
            n135 = call "Data Monitor.vi"("Data"=w344) -> ("Data Out"=w341:string, "Identifier"=w342:string)  [unwired: 9 in]
            n136 = in-place {
              in-place-border: w341 -> [w348]
              in-place-border: w340 -> [w347]
              n137 = in-place-map #9(w346, w342) -> (w350:T2)  [unwired: 1 in, 1 out]
              n138 = Bundle By Name(cluster=w350, "Data"=w348, "Source"=w347) -> (w349:T2)
              n139 = in-place-map #9(w349) -> (w345:map{string, T2})  [unwired: 1 in, 2 out]
            }
            n140 = in-place-cluster #8("Data"=w345) -> (w338:T6)
          }
        }
        n141 = Wait (ms)(milliseconds to wait=u32 500 ("等待时间（毫秒）")) -> ()  [unwired: 1 out]
        n142 = Unbundle By Name(w325) -> ("Data List"=w323:T2[], "Data"=w324:map{string, T2})
        n143 = for {
          tunnel: w324 -> [w335]
          tunnel: w323 -> [w332] mode=indexing
          tunnel: [w333] -> w321 mode=indexing
          n144 = Unbundle By Name(w332) -> ("Identifier"=w334:string)
          n145 = Look In Map(map=w335, key=w334) -> (value=w333:T2)  [unwired: 1 in, 1 out]
        }
        n146 = Bundle By Name(cluster=w325, "Data List"=w321) -> (w322:T6)
      }
      frame "Send" {
        n147 = Unbundle By Name(w352) -> ("Queue Ref.Name"=w355:string, "Type"=w358:map{string, string}, "Data"=w357:map{string, T2})
        n148 = for {
          tunnel: w357 -> [w370] mode=indexing
          shift-right: [w368] -> w354
          shift-left: w358 -> [w369]
          n149 = Unbundle By Name(w370) -> ("Data.Identifier"=w367:string, "Data.Data"=w366:string)
          n150 = Insert Into Map(map in=w369, key=w367, value=w366) -> (map out=w368:map{string, string})  [unwired: 2 out]
        }
        n151 = Unbundle By Name(w352) -> ("Queue Ref.Caller"=w351:refnum<queue>)
        n152 = Bundle("Name"=w355, "Type"=w354) -> (w353:T10)  [unwired: 1 in]
        n153 = call "Queue In.vi"("Data"=w353, "Message"="Read", "Queue In"=w351) -> ()  [unwired: 7 in, 2 out]
        n154 = Unbundle By Name(w352) -> ("Data"=w361:map{string, T2}, "Data List"=w356:T2[])
        n155 = for {
          tunnel: w361 -> [w374]
          tunnel: [w373] -> w360 mode=indexing
          tunnel: w356 -> [w372] mode=indexing
          n156 = Unbundle By Name(w372) -> ("Identifier"=w371:string)
          n157 = Look In Map(map=w374, key=w371) -> (value=w373:T2)  [unwired: 1 in, 1 out]
        }
        n158 = Bundle By Name(cluster=w352, "Data List"=w360) -> (w359:T6)
      }
      frame "====Driver====" {
      }
      frame "Open" {
        n159 = Unbundle By Name(w402) -> ("dll Path"=w379:path, "CAN.CANModel"=w397:u32, "CAN.Index"=w399:u32, "CAN.Reserved"=w398:u32, "CAN.CANChannel"=w396:u32, "CAN.TCPMode"=w387:u32, "CAN.RemotePort"=w386:u32, "CAN.LocalPort"=w385:u32, "CAN.IP"=w384:string)
        n160 = call "ZCAN_OpenDevice.vi"("dll Path"=w379, "reserved"=w398, "device_index"=w399, "device_type"=w397) -> ("error out"=w381:errorcluster, "DEVICE_HANDLE"=w382:u32)  [unwired: 5 in, 1 out]
        n161 = Bundle By Name(cluster=T8 {"tcp_type"=0, "work_port"=0, "local_port"=0, "IP"=""} ("ZCAN_InitCAN_setting_CANET"), "tcp_type"=w387, "work_port"=w386, "local_port"=w385, "IP"=w384) -> (w388:T8)
        n162 = call "Queue Clear.vi"("error in (no error)"=w405, "Filter"="Error,Exit", "Queue In"=w406) -> ("error out"=w404:errorcluster, "Queue Out"=w403:refnum<queue>)  [unwired: 7 in]
        n163 = call "ZCAN_InitCAN( CANET ).vi"("设备类型"=w397, "Dll Path"=w379, "device_hande"=w382, "CANindex"=w396, "ZCAN_InitCAN_setting_CANET"=w388, "error in (no error)"=w381) -> ("can_index_handle"=w393:u32, "error out"=w392:errorcluster)  [unwired: 8 in]
        n164 = call "ZCAN_StartCAN.vi"("error in (no error)"=w392, "can_index_handle"=w393, "Dll Path"=w379) -> ("error out"=w391:errorcluster, "can_index_handle(out)"=w380:u32, "startcan_success?"=w390:bool)  [unwired: 6 in]
        n165 = Not(x=w391) -> (.not. x?=w395:bool)
        n166 = And(x=w390, y=w395) -> (x .and. y?=w394:bool)
        n167 = case shown="真" w394 {
          tunnel: [w410 w416] -> w378
          tunnel: w402 -> [w410 w417]
          tunnel: ["Error,Close,Open" "Delay"] -> w401
          tunnel: [w408 _] -> w400
          tunnel: w382 -> [_ w414]
          tunnel: w391 -> [w408 _]
          tunnel: w380 -> [_ w413]
          frame False {
            n168 = Wait (ms)(milliseconds to wait=u32 500 ("等待时间（毫秒）")) -> ()  [unwired: 1 out]
          }
          frame True {
            n169 = Bundle By Name(cluster=w417, "CAN.DeviceRef"=w414, "CAN.ChannelRef"=w413, "Open?"=TRUE) -> (w416:T6)
          }
        }
        n170 = Unbundle By Name(w378) -> ("Open?"=→"Open":bool)
      }
      frame "Read" {
        n171 = Unbundle By Name(w419) -> ("CAN.Read?"=w418:bool)  [unwired: 1 out]
        n172 = case shown="真" w418 {
          tunnel: [_ w435] -> w424
          tunnel: [_ w434] -> w423
          tunnel: [w427 w433] -> w422
          tunnel: [_ w432] -> w421
          tunnel: w420 -> [_ w429]
          tunnel: w419 -> [w427 w428]
          frame False {
          }
          frame True {
            w431 = map{string, T2} {}  # Data
            n173 = flat-sequence {
              tunnel: [w441] -> w437
              tunnel: [w440] -> w436
              tunnel: w428 -> [w446]
              tunnel: w429 -> [w440]
              tunnel: w428 -> [w439]
              tunnel: [w465] -> w430
              tunnel: w437 -> [w465]
              tunnel: w436 -> [w463]
              frame #0 {
                n174 = Unbundle By Name(w446) -> ("dll Path"=w438:path, "CAN.ChannelRef"=w445:u32)
                n175 = call "ZCAN_Receive.vi"("dll Path"=w438, "can_handle"=w445) -> ("error out"=w442:errorcluster, "CAN数据帧数组"=w443:T11, "Receive_Num"=w444:u32)  [unwired: 3 in]
                n176 = case shown="1.." w444 {
                  tunnel: w443 -> [_ w458]
                  tunnel: w442 -> [w447 w457]
                  tunnel: [w447 w456] -> w441
                  tunnel: w439 -> [_ w451]
                  frame 0, Default {
                  }
                  frame 1.. {
                    n177 = Unbundle By Name(w451) -> ("Queue Ref.Caller"=w450:refnum<queue>, "CAN Fram"=w449:map{string, map{string, T4}})
                    n178 = call "ParsesCANFrame.vi"("error in (no error)"=w457, "CAN Fram"=w449, "CAN数据帧数组"=w458) -> ("error out"=w456:errorcluster, 1:"Data Out"=→"Read":string[][], 3:"Data Out"=→"Receive Frame":string, "Data"=w452:string[], "Write?"=w448:bool, "ID"=w453:string[])  [unwired: 1 in, 2 out]
                    n179 = case shown="真" w448 {
                      tunnel: w453 -> [_ w461]
                      tunnel: w452 -> [_ w460]
                      tunnel: w450 -> [_ w459]
                      frame False {
                      }
                      frame True {
                        n180 = call "000_Source Write.vim"("Data"=w460, "Name"=w461, "Queue In"=w459) -> ()  [unwired: 6 in, 3 out]
                      }
                    }
                  }
                }
              }
              frame #1 {
                n181 = Tick Count (ms)() -> (millisecond timer value=w464:u32)
                n182 = Subtract(x=w464, y=w463) -> (x-y=→"Read Delay(ms)":u32)
              }
            }
            n183 = Bundle By Name(cluster=w428, "Data"=w431) -> (w433:T6)
            n184 = case shown="错误 .." w430 {
              selector: w430 -> [_ w466]
              tunnel: [_ "Error,Open"] -> w435
              tunnel: [_ TRUE] -> w434
              tunnel: w433 -> [_ _]
              tunnel: [_ w466] -> w432
              frame No Error {
              }
              frame Error {
              }
            }
          }
        }
      }
      frame "Refresh List" {
        n185 = Unbundle By Name(w471) -> ("All Data"=w470:string[][], "Data"=w469:map{string, T2})
        n186 = for {
          tunnel: w470 -> [w491] mode=indexing
          tunnel: w469 -> [w492]
          tunnel: [w476] -> _ mode=indexing
          n187 = Index Array(array=w491) -> (element=w490:string)  [unwired: 1 in]
          n188 = Look In Map(map=w492, key=w490) -> (value=w489:T2)  [unwired: 1 in, 1 out]
          n189 = Unbundle By Name(w489) -> ("Identifier"=w488:string, "Name"=w487:string, "Address"=w486:string, "Unit"=w485:string, "Lower"=w483:dbl, "Upper"=w480:dbl, "Set Value"=w478:string, "Formula"=w477:string, "Data"=w475:string)
          n190 = Format Into String(format string="%#.3f" ("格式字符串"), w483) -> (resulting string=w482:string)  [unwired: 2 in, 1 out]
          n191 = Format Into String(format string="%#.3f" ("格式字符串"), w480) -> (resulting string=w479:string)  [unwired: 2 in, 1 out]
          n192 = Build Array(w488, w487, w486, w485, w482, w479, w478, w477, w475) -> (w476:string[])
        }
      }
      frame "Write" {
        n193 = Unbundle By Name(w499) -> ("CAN Element"=w500:u8[], "ZCAN_Transmit_Data"=w501:T5, "CAN Fram"=w502:map{string, map{string, T4}}, "Queue Ref.Project Name"=w503:string, "CAN.Write?"=w495:bool)
        n194 = case shown="真" w495 {
          tunnel: w503 -> [_ w527]
          tunnel: w502 -> [_ w526]
          tunnel: w501 -> [_ w525]
          tunnel: w500 -> [_ w523]
          tunnel: w499 -> [w509 w514]
          tunnel: [TRUE w518] -> w498
          tunnel: [_ w517] -> w497
          tunnel: [_ w515] -> _
          tunnel: [w509 w512] -> w494
          tunnel: "ID" -> [_ w513]
          frame False {
          }
          frame True {
            n195 = call "Data Global.vi"("Name"=w527) -> ("Data Out"=w524:map{string, T2})  [unwired: 7 in, 3 out]
            n196 = for {
              tunnel: w526 -> [w557] mode=indexing
              tunnel: w525 -> [w562]
              tunnel: w524 -> [w561]
              tunnel: w523 -> [w559]
              tunnel: [w542] -> w521 mode=indexing if=w528
              tunnel: [w539] -> w516 mode=indexing if=w528
              tunnel: [w536] -> w515 mode=indexing
              shift-right: [w531] -> w512
              shift-left: w514 -> [w532]
              tunnel: w513 -> [w530]
              w555 = u8 0
              n197 = Unbundle By Name(w557) -> ("CAN Data"=w560:map{string, T4})
              n198 = for {
                tunnel: w561 -> [w584]
                tunnel: w560 -> [w578] mode=indexing
                shift-right: [w573] -> w537
                shift-left: w559 -> [w583]
                tunnel: [w567] -> w540
                shift-right: [w577] -> w531
                shift-left: w532 -> [w577]
                tunnel: w530 -> [w575]
                tunnel: [w566] -> w529
                n199 = Unbundle By Name(w578) -> ("CAN.CAN Byte Offset"=w580:i32, "CAN.CAN Bit Offset"=w581:i32, "CAN.Type"=w572:string, "CAN.ID"=w576:string)
                n200 = Unbundle By Name(w578) -> ("CAN.Write Enable"=w566:bool, "CAN.CAN Message ID"=w567:string)
                n201 = Look In Map(map=w584, key=w576) -> (value=w582:T2)  [unwired: 1 in, 1 out]
                n202 = Equal?(x=w576, y=w575) -> (x = y?=w574:bool)
                n203 = Unbundle By Name(w582) -> ("Data"=w579:string)
                n204 = case shown="\"bool\"" w572 {
                  tunnel: w583 -> [w592 w597 w613 w618 w628 w635]
                  tunnel: [w592 w596 w612 w621 w633 w640] -> w573
                  tunnel: w581 -> [_ w595 _ _ _ _]
                  tunnel: w580 -> [_ w594 w611 w620 w632 w639]
                  tunnel: w579 -> [_ w593 w608 w617 w627 w634]
                  tunnel: [_ _ _ w615 _ _] -> w571
                  tunnel: [_ _ _ w617 _ _] -> w570
                  tunnel: [_ _ _ w616 _ _] -> w569
                  tunnel: [_ _ _ w614 _ _] -> w568
                  frame Default {
                  }
                  frame "bool" {
                    n205 = in-place {
                      in-place-border: w595 -> [w602]
                      in-place-border: w593 -> [w599]
                      n206 = in-place-array #10(w597, w594) -> (w606:u8)
                      n207 = To Lower Case(string=w599) -> (all lower case string=w601:string)
                      n208 = case shown="\"1\", \"true\"" w601 {
                        tunnel: [_ TRUE] -> w600
                        frame Default {
                        }
                        frame "1", "true" {
                        }
                      }
                      n209 = Number To Boolean Array(number=w606) -> (Boolean array=w605:bool[])
                      n210 = Replace Array Subset(array=w605, new element=w600, index=w602) -> (w604:bool[])
                      n211 = Boolean Array To Number(Boolean array=w604) -> (number=w603:u32)
                      n212 = To Unsigned Byte Integer(number=w603) -> (unsigned 8bit integer=w598:u8)
                      n213 = in-place-array #10(w598) -> (w596:u8[])  [unwired: 1 out]
                    }
                  }
                  frame "byte" {
                    n214 = Fract/Exp String To Number(string=w608, default (0 dbl)=u8 0 ("默认(0 DBL)")) -> (number=w609:u8)  [unwired: 2 in, 1 out]
                    n215 = Replace Array Subset(array=w613, new element=w609, index=w611) -> (w612:u8[])
                  }
                  frame "dword" {
                    n216 = Fract/Exp String To Number(string=w617, default (0 dbl)=u32 0 ("默认(0 DBL)")) -> (number=w616:u32)  [unwired: 2 in, 1 out]
                    n217 = Type Cast(type=w618, x=w616) -> (*(type *) &x=w615:u8[])
                    n218 = for {
                      tunnel: w615 -> [w623] mode=indexing
                      tunnel: [w622] -> w614 mode=indexing
                      n219 = Format Into String(format string="%02x " ("格式字符串"), w623) -> (resulting string=w622:string)  [unwired: 2 in, 1 out]
                    }
                    n220 = Replace Array Subset(array=w618, new element=w615, index=w620) -> (w621:u8[])
                  }
                  frame "float" {
                    n221 = Fract/Exp String To Number(string=w627, default (0 dbl)=sgl 0.0 ("默认(0 DBL)")) -> (number=w630:sgl)  [unwired: 2 in, 1 out]
                    n222 = expression code="x*1000"(w630) -> (w626:sgl)
                    n223 = To Unsigned Long Integer(number=w626) -> (unsigned 32bit integer=w625:u32)
                    n224 = Type Cast(type=w628, x=w625) -> (*(type *) &x=w629:u8[])
                    n225 = Replace Array Subset(array=w628, new element=w629, index=w632) -> (w633:u8[])
                  }
                  frame "word" {
                    n226 = Fract/Exp String To Number(string=w634, default (0 dbl)=u16 0 ("默认(0 DBL)")) -> (number=w637:u16)  [unwired: 2 in, 1 out]
                    n227 = Type Cast(type=w635, x=w637) -> (*(type *) &x=w636:u8[])
                    n228 = Replace Array Subset(array=w635, new element=w636, index=w639) -> (w640:u8[])
                  }
                }
                n229 = case shown="真" w574 {
                  tunnel: [_ w591] -> _
                  tunnel: w573 -> [_ w591]
                  tunnel: w572 -> [_ w590]
                  tunnel: [_ w590] -> _
                  tunnel: [_ w589] -> _
                  tunnel: w571 -> [_ w589]
                  tunnel: [_ w588] -> _
                  tunnel: w570 -> [_ w588]
                  tunnel: w569 -> [_ w587]
                  tunnel: [_ w587] -> _
                  tunnel: [_ w586] -> _
                  tunnel: w568 -> [_ w586]
                  tunnel: [_ w585] -> _
                  tunnel: w567 -> [_ w585]
                  frame False {
                  }
                  frame True {
                  }
                }
              }
              n230 = Array Size(array=w537) -> (size(s)=w536:i32)
              n231 = Not(x=w529) -> (.not. x?=w528:bool)
              n232 = Array To Cluster(array=w537) -> (cluster=w556:T12)
              n233 = Scan From String(format string="0X%x" ("格式字符串"), input string=w540) -> (output 1=w534:u32)  [unwired: 3 in, 3 out]
              n234 = for {
                tunnel: w537 -> [w564] mode=indexing
                tunnel: [w563] -> w538 mode=indexing
                n235 = Format Into String(format string="%02x " ("格式字符串"), w564) -> (resulting string=w563:string)  [unwired: 2 in, 1 out]
              }
              n236 = Bundle By Name(cluster=w562, "DATA"=w556, "ID"=w534) -> (w543:T5)
              n237 = Unbundle(w543) -> ("帧类型"=w549:u32, "帧格式"=w548:u32, "ID"=w547:u32, "数据长度"=w546:u8, "DATA"=w545:T13, "发送方式"=w544:u32)
              n238 = Concatenate Strings(w538) -> (w541:string)
              n239 = Format Into String(format string="0x%02x " ("格式字符串"), w534) -> (resulting string=w533:string)  [unwired: 2 in, 1 out]
              n240 = Logical Shift(y=i16 30, x=w548) -> (x << y=w551:u32)
              n241 = Logical Shift(y=i16 31, x=w549) -> (x << y=w554:u32)
              n242 = Compound Arithmetic op=OR ("复合运算")(w554, w551, w547) -> (w550:u32)
              n243 = Build Array(w533, w541) -> (w539:string[])
              n244 = Bundle ("捆绑")(w550, "数据长度"=w546, w555, w555, w555, "DATA"=w545, "发送方式"=w544) -> (w542:T14)  [unwired: 1 in]
            }
            "Write" <- w516
            n245 = Unbundle By Name(w514) -> ("CAN.ChannelRef"=w522:u32)
            n246 = Unbundle By Name(w512) -> ("dll Path"=w511:path)
            n247 = Array Size(array=w521) -> (size(s)=w519:i32)
            n248 = dll-call lib="D:/NBT/Code/V3.1/NBT-TestPlatform 20230705_1/Data/zlgcan_wrap.dll" fn="ZCAN_Transmit"(path in=w511, "通道句柄"=w522, "数据帧数组"=w521, "数据帧数"=w519) -> (error out=w517:errorcluster, "返回类型"=w520:u32)  [unwired: 5 in, 1 out]
            n249 = Equal?(x=w520, y=w519) -> (x = y?=w518:bool)
          }
        }
        n250 = case shown="真" w498 {
          tunnel: ["Error,Close,Open" _] -> w506
          tunnel: [TRUE _] -> w505
          tunnel: [w641 _] -> w504
          tunnel: w497 -> [w643 _]
          tunnel: w496 -> [_ w647]
          frame False {
            n251 = Merge Errors(w643, errorcluster {"status"=TRUE, "code"=5100, "source"="CAN发送失败"} ("error out")) -> (w641:errorcluster)
          }
          frame True {
            n252 = Tick Count (ms)() -> (millisecond timer value=w648:u32)
            n253 = Subtract(x=w648, y=w647) -> (x-y=→"Write Delay(ms)":u32)
          }
        }
      }
      frame "Write Test" {
        n254 = Unbundle By Name(w656) -> ("CAN Element"=w650:u8[], "ZCAN_Transmit_Data"=w657:T5, "Queue Ref.Project Name"=w658:string, "Open?"=w652:bool)
        n255 = Type Cast(type=w650, x="Multiple Parameter") -> (*(type *) &x=w649:u8[])
        n256 = case shown="真" w652 {
          tunnel: w658 -> [_ _]
          tunnel: w657 -> [_ w691]
          tunnel: w656 -> [w667 w690]
          tunnel: [TRUE w686] -> w655
          tunnel: [_ w685] -> w654
          tunnel: w649 -> [_ w675]
          frame False {
            n257 = Unbundle By Name(w667) -> ("Queue Ref.UI"=w666:refnum<queue>)
            n258 = call "Queue In.vi"("Data"="设备未连接，请检查网络和配置！", "Message"="PopUp", "Queue In"=w666) -> ()  [unwired: 7 in, 2 out]
          }
          frame True {
            w683 = 8 ("y")
            n259 = Array Size(array=w675) -> (size(s)=w684:i32)
            n260 = Quotient & Remainder(x=w684, y=w683) -> (x-y*floor(x/y)=w682:i32, floor(x/y)=w678:i32)
            n261 = Greater Than 0?(x=w682) -> (x > 0?=w681:bool)
            n262 = Select(t=1 ("维数大小"), s=w681, f=0 ("维数大小")) -> (s? t:f=w677:i32)
            n263 = Add(x=w677, y=w678) -> (x+y=w676:i32)
            n264 = Reshape Array(w675, w676, w683) -> (w674:u8[][])
            n265 = for {
              tunnel: w691 -> [w723]
              tunnel: [w709] -> w688 mode=indexing
              tunnel: [w707] -> w673 mode=indexing
              tunnel: w674 -> [w702] mode=indexing
              tunnel: "Start Frame" -> [w701]
              i -> [w700]
              w722 = u8 0
              n266 = Array To Cluster(array=w702) -> (cluster=w703:T12)
              n267 = Add(x=w701, y=w700) -> (x+y=w699:u32)
              n268 = Bundle By Name(cluster=w723, "DATA"=w703, "ID"=w699) -> (w710:T5)
              n269 = for {
                tunnel: [w725] -> w706 mode=indexing
                tunnel: w702 -> [w724] mode=indexing
                n270 = Format Into String(format string="%02x " ("格式字符串"), w724) -> (resulting string=w725:string)  [unwired: 2 in, 1 out]
              }
              n271 = Unbundle(w710) -> ("帧类型"=w716:u32, "帧格式"=w715:u32, "ID"=w714:u32, "数据长度"=w713:u8, "DATA"=w712:T13, "发送方式"=w711:u32)
              n272 = Concatenate Strings(w706) -> (w708:string)
              n273 = Format Into String(format string="0x%02x " ("格式字符串"), w699) -> (resulting string=w704:string)  [unwired: 2 in, 1 out]
              n274 = Logical Shift(y=i16 30, x=w715) -> (x << y=w718:u32)
              n275 = Logical Shift(y=i16 31, x=w716) -> (x << y=w721:u32)
              n276 = Compound Arithmetic op=OR ("复合运算")(w721, w718, w714) -> (w717:u32)
              n277 = Build Array(w704, w708) -> (w707:string[])
              n278 = Bundle ("捆绑")(w717, "数据长度"=w713, w722, w722, w722, "DATA"=w712, "发送方式"=w711) -> (w709:T14)  [unwired: 1 in]
            }
            "Write Test" <- w673
            n279 = Unbundle By Name(w690) -> ("dll Path"=w669:path, "CAN.ChannelRef"=w689:u32)
            n280 = Array Size(array=w688) -> (size(s)=w671:i32)
            n281 = Greater Than 0?(x=w671) -> (x > 0?=w670:bool)
            n282 = case shown="真" w670 {
              tunnel: w689 -> [_ w698]
              tunnel: w688 -> [_ w697]
              tunnel: [w692 w696] -> w687
              tunnel: [_ w695] -> w685
              tunnel: w671 -> [w692 w694]
              tunnel: w669 -> [_ w693]
              frame False {
              }
              frame True {
                n283 = dll-call lib="D:/NBT/Code/V3.1/NBT-TestPlatform 20230705_1/Data/zlgcan_wrap.dll" fn="ZCAN_Transmit"(path in=w693, "通道句柄"=w698, "数据帧数组"=w697, "数据帧数"=w694) -> (error out=w695:errorcluster, "返回类型"=w696:u32)  [unwired: 5 in, 1 out]
              }
            }
            n284 = Equal?(x=w687, y=w671) -> (x = y?=w686:bool)
          }
        }
        n285 = case shown="真" w655 {
          tunnel: ["Error,Close,Open" _] -> w661
          tunnel: [TRUE _] -> w660
          tunnel: [w727 _] -> w659
          tunnel: w654 -> [w729 _]
          tunnel: w653 -> [_ _]
          frame False {
            n286 = Merge Errors(w729, errorcluster {"status"=TRUE, "code"=5100, "source"="CAN发送失败"} ("error out")) -> (w727:errorcluster)
          }
          frame True {
          }
        }
      }
      frame "Close" {
        n287 = Unbundle By Name(w739) -> ("dll Path"=w732:path, "CAN.DeviceRef"=w737:u32, "CAN.ChannelRef"=w738:u32)
        n288 = Greater Than 0?(x=w738) -> (x > 0?=w736:bool)
        n289 = case shown="真" w736 {
          tunnel: w738 -> [_ w745]
          tunnel: w737 -> [_ w744]
          tunnel: w732 -> [_ w742]
          frame False {
          }
          frame True {
            n290 = call "ZCAN_ResetCAN.vi"("can_handle"=w745, "Path"=w742) -> ("error out"=w746:errorcluster)  [unwired: 8 in, 1 out]
            n291 = call "ZCAN_CloseDevice.vi"("error in (no error)"=w746, "device_handle"=w744, "路径输入"=w742) -> ("error out"=w743:errorcluster)  [unwired: 7 in, 1 out]
            n292 = call <vilib>:"Clear Errors.vi"("error in (no error)"=w743) -> ()  [unwired: 5 in, 2 out]
          }
        }
        n293 = Bundle By Name(cluster=w739, "CAN.DeviceRef"=u32 0 ("CAN.Device Ref"), "CAN.ChannelRef"=u32 0 ("CAN.Channel Ref")) -> (w735:T6)
      }
      frame "Delay" {
        n294 = Unbundle By Name(w749) -> ("Delay.Next"=w753:string, "Delay.Count Time(ms)"=w750:u32, "Delay.Delay Time(ms)"=w751:u32)
        n295 = call "Delay Judge.vi"("Delay Time(ms)"=w751, "Count Time(ms)"=w750) -> ("Time Out?"=w752:bool)  [unwired: 5 in, 4 out]
        n296 = Select(t=w753, s=w752, f=w748) -> (s? t:f=w747:string)
      }
      frame "Error" {
        n297 = Unbundle By Name(w760) -> ("Queue Ref.Data Path"=w759:path, "Queue Ref.Name"=w757:string)
        n298 = call "000 Write Error.vi"("Data"=w758, "Name"=w757, "Path"=w759) -> ("Error"=→"Error":string)  [unwired: 7 in, 1 out]
      }
      frame "Exit" {
        n299 = call "Queue Clear.vi"("error in (no error)"=w765, "Queue In"=w767) -> ("error out"=w764:errorcluster, "Queue Out"=w766:refnum<queue>)  [unwired: 8 in]
      }
      frame "Quit" {
      }
    }
    n300 = call "Queue In.vi"("First"=w28, "error in (no error)"=w33, "Data"=w31, "Message"=w32, "Queue In"=w36) -> ("error out"=w34:errorcluster, "Queue Out"=w35:refnum<queue>)  [unwired: 5 in]
  }
  n301 = while {
    tunnel: w13 -> [w776]
    tunnel: [w774] -> w14
    tunnel: w2 -> [w773]
    stop <- w775 stop-if-true
    n302 = event shown="[1] 键按下" {
      selector: w776 -> [_ _ _ _ _ _ _]
      dyn-events: [_ _ _ _ _ _ _] -> w774
      timeout: _ -> [_ _ _ _ _ _ _]
      tunnel: [_ _ _ _ w790 _ _] -> w775
      tunnel: w773 -> [_ w781 w786 w789 _ w794 w805]
      event Timeout {
        n303 = event-data() -> ()  [unwired: 1 in, 1 out]
      }
      event Key Down {
        n304 = event-data() -> ("Char"=w780:i16, "VKey"=w779:T15, "Mods"=w778:cluster{"Num Pad":bool, "Menu Key":bool}, "PlatMods"=w777:T16)  [unwired: 1 in]
        n305 = call "Queue Key Down.vi"("Queue Ref Out"=w781, "C"=w780, "Platform Key"=w777, "Group Key"=w778, "V Key"=w779) -> ()  [unwired: 6 in, 1 out]
      }
      event "Data Load", "Write Test": Value Change {
        n306 = event-data() -> ("CtlRef"=w785:refnum<vi>)  [unwired: 1 in]
        n307 = property class="Bool"(reference=w785) -> ("Label.Text"=w784:string)  [unwired: 1 in, 2 out]
        n308 = Unbundle By Name(w786) -> ("Data"=w783:refnum<queue>)
        n309 = call "Queue In.vi"("First"=TRUE, "Message"=w784, "Queue In"=w783) -> ()  [unwired: 7 in, 2 out]
      }
      event Panel Resize {
        n310 = event-data() -> ()  [unwired: 1 in, 1 out]
        n311 = Unbundle By Name(w789) -> ("Message"=w788:refnum<queue>)
        n312 = call "Queue In.vi"("Message"="Panel Change", "Queue In"=w788) -> ()  [unwired: 8 in, 2 out]
      }
      event User Event {
        n313 = event-data() -> ("Message"=w792:string)  [unwired: 1 in]
        n314 = Equal?(x=w792, y="Exit") -> (x = y?=w790:bool)
      }
      event Panel Close? {
        n315 = event-data() -> ()  [unwired: 1 in, 1 out]
        n316 = Unbundle By Name(w794) -> ("Message"=w793:refnum<queue>)
        n317 = Call Chain() -> (call chain=w797:string[])
        n318 = Array Size(array=w797) -> (size(s)=w796:i32)
        n319 = case shown="0, 默认" w796 {
          tunnel: ["Exit Prepare" ("Message") "Panel Hidden" ("Message")] -> w795
          frame 0, Default {
          }
          frame 2.. {
          }
        }
        n320 = call "Queue In.vi"("Message"=w795, "Queue In"=w793) -> ()  [unwired: 8 in, 2 out]
        n321 = event-data("Discard?"=TRUE ("放弃？")) -> ()  [unwired: 1 in, 1 out]
      }
      event "CAN Enable": Value Change {
        n322 = event-data() -> ("CtlRef"=w803:refnum<vi>)  [unwired: 1 in]
        n323 = Unbundle By Name(w805) -> ("Data"=w804:refnum<queue>)
        n324 = property class="Bool (严格)"(reference=w803) -> ("Label.Text"=w802:string)  [unwired: 1 in, 2 out]
        n325 = call "Queue In.vi"("Data"="CAN Enable", "Message"=w802, "Queue In"=w804) -> ()  [unwired: 7 in, 2 out]
      }
    }
  }
  n326 = while {
    tunnel: w18 -> [w815]
    tunnel: [w812] -> w16
    tunnel: [w811] -> w17
    tunnel: w2 -> [w808]
    shift-right: [w807] -> _
    shift-left: _ -> [w806]
    stop <- w819 stop-if-true
    n327 = call "Queue Out.vi"("Queue In"=w815) -> ("error out"=w818:errorcluster, "Data"=w816:variant, "Message"=w817:string, "Queue Out"=w814:refnum<queue>)  [unwired: 6 in, 1 out]
    n328 = case shown="\"Panel Change\"" w817 {
      selector: w817 -> [_ _ _ _ _ _ _ _ w861 _]
      tunnel: w814 -> [w822 w828 w834 w838 w846 w852 w855 w858 w868 w875]
      tunnel: w818 -> [w821 w827 w833 w837 w845 w851 w854 w857 w866 w876]
      tunnel: [w822 w828 w834 w838 w846 w852 w855 w858 w867 w875] -> w813
      tunnel: [w821 w827 w833 w837 w845 w851 w854 w857 w865 w876] -> w810
      tunnel: [_ "Panel Change" _ _ _ _ _ _ "Quit" _] -> w809
      tunnel: [_ _ _ _ _ _ _ _ _ TRUE] -> w819
      tunnel: w816 -> [_ _ w831 w835 w842 _ _ _ _ _]
      tunnel: w808 -> [_ w823 _ _ _ _ _ _ _ _]
      tunnel: [w820 w824 w832 w836 w843 w850 w853 w856 w860 w873] -> w807
      tunnel: w806 -> [w820 _ w832 w836 w844 w850 w853 w856 w860 w873]
      frame "eee", Default {
      }
      frame "Init" {
        n329 = Bundle By Name(cluster=T17 {"Queue List"={}, "Active Panel"="", "Queue"={"UI"=refnum, "Message"=refnum, "Data"=refnum, "Caller"=refnum, "Name"="", "Data Path"=path "", "Class Path"=path "", "SubPanel"=refnum, "Project Name"="", "MNT"="", "Title"="", "Data Source"=refnum, "Queue List"={}, "VI"=refnum, "UE"=refnum}, "Active Row"=0, "All Data"=[]}, "Queue"=w823) -> (w824:T17)
      }
      frame "PopUp" {
        n330 = Variant To Data(type="", Variant=w831) -> (data=w829:string)  [unwired: 1 in, 1 out]
        n331 = One Button Dialog(message=w829) -> ()  [unwired: 1 in, 1 out]
      }
      frame "Refresh Class Ref" {
        n332 = in-place {
          in-place-border: w835 -> [w841]
          n333 = in-place-cluster #11(w836) -> ("Queue"=w840:T1)
          n334 = Variant To Data(type=w840, Variant=w841) -> (data=w839:T1)  [unwired: 1 in, 1 out]
          n335 = in-place-cluster #11("Queue"=w839) -> ()  [unwired: 1 out]
        }
      }
      frame "Data Change" {
        n336 = in-place {
          in-place-border: w842 -> [w849]
          n337 = in-place-cluster #12(w844) -> ("All Data"=w848:string[][])
          n338 = Variant To Data(type=w848, Variant=w849) -> (data=w847:string[][])  [unwired: 1 in, 1 out]
          n339 = in-place-cluster #12("All Data"=w847) -> (w843:T17)
        }
      }
      frame "====System====" {
      }
      frame "Panel Change" {
        n340 = call "MCList Adjust.vi"() -> ()  [unwired: 11 in, 1 out]
      }
      frame "====User====" {
      }
      frame "Exit" {
        n341 = Unbundle By Name(w860) -> ("Queue.UE"=w859:refnum<user-event>, "Queue.Message"=w864:refnum<queue>, "Queue.Data"=w863:refnum<queue>)
        n342 = Build Array(w864, w863) -> (w862:refnum<queue>[])
        n343 = for {
          tunnel: w862 -> [w872] mode=indexing
          tunnel: w861 -> [w871]
          n344 = call "Queue In.vi"("First"=TRUE, "Message"=w871, "Queue In"=w872) -> ()  [unwired: 7 in, 2 out]
        }
        n345 = Generate User Event(user event=w859, event data cluster=w861) -> ()  [unwired: 2 in, 2 out]
        n346 = call "Queue Clear.vi"("error in (no error)"=w866, "Queue In"=w868) -> ("error out"=w865:errorcluster, "Queue Out"=w867:refnum<queue>)  [unwired: 8 in]
      }
      frame "Quit" {
      }
    }
    n347 = call "Queue In.vi"("error in (no error)"=w810, "Message"=w809, "Queue In"=w813) -> ("error out"=w811:errorcluster, "Queue Out"=w812:refnum<queue>)  [unwired: 7 in]
  }
  n348 = call "000 Driver Message.vi"("Queue In"=w2) -> ("error out"=w24:errorcluster)  [unwired: 8 in, 2 out]
  n349 = call "Queue Release.vi"("error in (no error)"=w6, "Queue In"=w5) -> ("error out"=w25:errorcluster)  [unwired: 9 in]
  n350 = call "Queue Release.vi"("error in (no error)"=w17, "Queue In"=w16) -> ("error out"=w20:errorcluster)  [unwired: 9 in]
  n351 = Unregister For Events(event registration refnum=w14) -> (error out=w15:errorcluster)  [unwired: 1 in]
  n352 = Destroy User Event(user event=w12, error in=w15) -> (error out=w19:errorcluster)
  n353 = Call Chain() -> (call chain=w22:string[])
  n354 = Merge Errors(w19, w20, w24, w25) -> (w21:errorcluster)
  n355 = Array Size(array=w22) -> (size(s)=w23:i32)
  n356 = case shown="2.." w23 {
    tunnel: w21 -> [_ w877]
    frame 0, Default {
    }
    frame 2.. {
      n357 = invoke class="VI" method="FP.Close"(error in=w877) -> ()  [unwired: 2 in, 3 out]
    }
  }
